vi "Register Track.vi"(6 "Track ID":u64, 7 "Track Name":string, 8 "error in":errorcluster) -> (0 "error out":errorcluster, 4 "Track ID":u64)   [LabVIEW 2027, in "VS Tracing API.lvlib"]
doc: "Creates a custom track that can be used for recording events outside timed structures.\nThe created track appears as a separate timeline in the trace and can be used with <i>Event Start On Track</i> and <i>Event Stop On Track</i>.\n\n<b>Parameters</b>\n• <b>Track Name</b>: Display name of the track shown in trace.\n• <b>Track ID</b>: User-defined unique identifier for the track.\n • If a non-zero value is provided, that value is used as the track identifier.\n • If not provided, or if set to 0, a unique track identifier is automatically generated.\n<b>Returns</b>\n• <b>Track ID</b>: Unique identifier assigned to the track. Use this value when recording events on the track through <i>Event Start On Track</i> and <i>Event Stop On Track</i>. \n\n<b>Notes</b>\n• The Track ID can be any user-defined unique value.\n• A track must be registered before events can be recorded on it."
uses:
  VS Tracing API.lvlib
  libvs_perfetto.dll
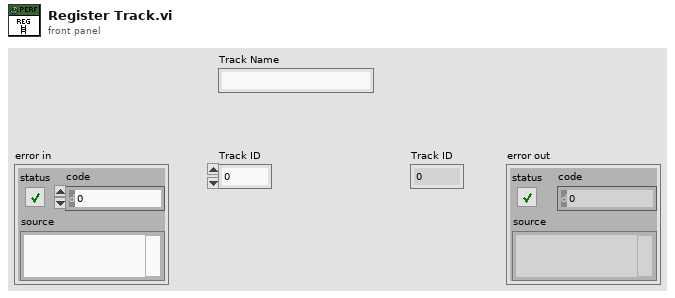
[diagram p1: front panel]
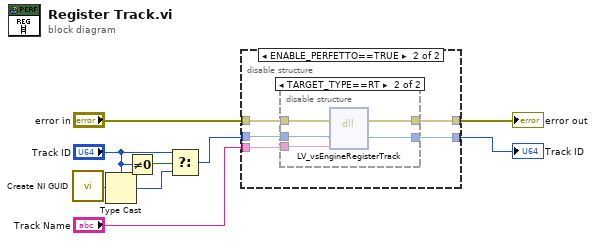
[diagram p0: block diagram]
diagram:
  n1 = call <vilib>:"Create NI GUID.vi"() -> ("NI GUID"=w6:string)
  n2 = Type Cast(type="Track ID", x=w6) -> (*(type *) &x=w3:u64)
  n3 = Not Equal To 0?(x="Track ID") -> (x != 0?=w4:bool)
  n4 = Select(t="Track ID", s=w4, f=w3) -> (s? t:f=w2:u64)
  n5 = disable-structure shown="ENABLE_PERFETTO==TRUE" {
    disable-tunnel: "Track Name" -> [_ w14]
    disable-tunnel: "error in" -> [w11 w15]
    disable-tunnel: [w11 w16] -> w8
    disable-tunnel: w2 -> [w10 w13]
    disable-tunnel: [w10 w12] -> w5
    frame condition #0 (active) {
    }
    frame condition #1 {
      n6 = disable-structure shown="TARGET_TYPE==RT" {
        disable-tunnel: [w18 w23] -> w16
        disable-tunnel: w15 -> [w18 w22]
        disable-tunnel: w14 -> [_ w21]
        disable-tunnel: w13 -> [w17 w20]
        disable-tunnel: [w17 w19] -> w12
        frame condition #0 (active) {
        }
        frame condition #1 {
          n7 = dll-call lib="libvs_perfetto.*" fn="LV_vsEngineRegisterTrack"(error in=w22, "trackId"=w20, "trackName"=w21) -> (error out=w23:errorcluster, "trackId"=w19:u64)  [unwired: 4 in, 1 out]
        }
      }
    }
  }
  "error out" <- w8
  "Track ID" <- w5
